vi "Acknowledge Execution.vi"(8 "error in (no error)":errorcluster, 10 "VI Refnum":refnum<vi>, 11 "Async Methods Actor in":refnum<class "Async Methods Actor.lvclass">) -> (0 "error out":errorcluster, 3 "Async Methods Actor out":refnum<class "Async Methods Actor.lvclass">)   [LabVIEW 2021, in "Async Methods Actor.lvlib" / "Async Methods Actor.lvclass"]
uses:
  Async Methods Actor.lvclass
  <vilib>/ActorFramework/Actor/Actor.lvclass
  Async Methods Actor Messages/Async Message/Async Message.lvclass
  Async Methods Actor.lvclass/Async Methods Actor.ctl
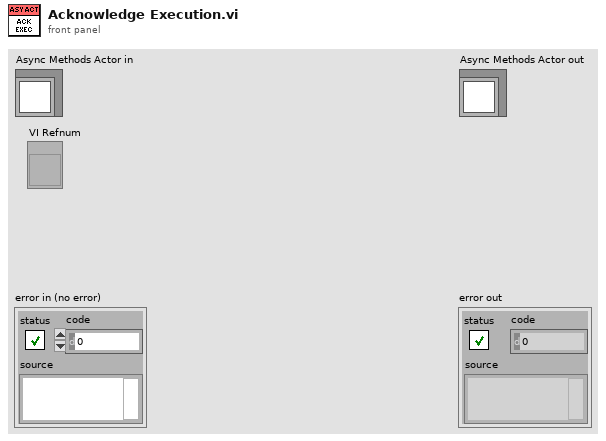
[diagram p1: front panel]
types:
  T1 = typedef "Async Methods Actor.lvlib/Async Methods Actor.lvclass/VI Refnums Map.ctl" = map{refnum<vi>, T2}
  T2 = typedef "Async Methods Actor.lvlib/Async Methods Actor.lvclass/VI Refnums Map Value.ctl" = cluster{"Async Call Method":T3, "Message Path":path}
  T3 = typedef "Async Methods Actor.lvlib/Async Methods Actor.lvclass/Async Call Method.ctl" = enum16{"Call and Collect", "Call and Forget"}
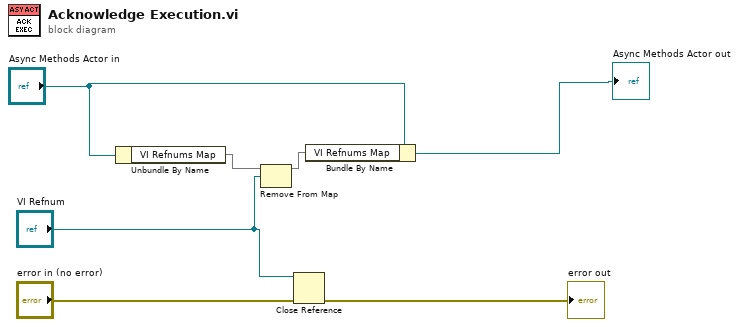
[diagram p0: block diagram]
diagram:
  n1 = Unbundle By Name("Async Methods Actor in") -> ("VI Refnums Map"=w7:T1)
  n2 = Remove From Map(10:"VI Refnum", 11:w7) -> (3:w6:T1)  [unwired: 2 out]
  n3 = Close Reference(reference="VI Refnum", error in (no error)="error in (no error)") -> (error out=→"error out":errorcluster)
  n4 = Bundle By Name(cluster="Async Methods Actor in", "VI Refnums Map"=w6) -> (→"Async Methods Actor out":refnum<class "Async Methods Actor.lvclass">)
